vi "general_testing.vi"() -> ()   [LabVIEW 2020]
uses:
  C:/Users/359167/Documents/LabVIEW_ws/Thorlabs.MotionControl.FTD2xx_Net.dll
  Thorlabs.MotionControl.FTD2xx_Net.dll
  <vilib>/DAQmx/create/channels.llb/DAQmx Create Channel (AI-Voltage-Basic).vi
  <vilib>/Utility/file.llb/Read Delimited Spreadsheet (DBL).vi
  <vilib>/Utility/file.llb/Write Delimited Spreadsheet (DBL).vi
  <resource>/objmgr/daqmx.rc
panel:
  out "Numeric 4":dbl
  in  "Numeric 3":dbl format="%#_13g"
  out "Numeric 2":dbl
  out "appended array":dbl[](array[numeric])
  in  "y":dbl
  out "all rows":dbl[][](array[numeric])
  in  "stop":bool
  out "Numeric":i16
  in  "Y":bool[](array[boolean])
  in  "X":bool[](array[boolean])
  out "Array":refnum<k21>[][](array[refnum])
  in  "input terminal configuration":i32(ring)=-1 items=["Default"=-1, "RSE"=10083, "NRSE"=10078, "Differential"=10106, "Pseudodifferential"=12529]
  in  "Cluster":T1
  out "mounts":string[](array[string])
  out "# of mounts":dbl
  in  "# of Channels":i32=4
  out "Y":dbl[](array[numeric])
  out "X":dbl[](array[numeric])
  out "Serial Number":string[](array[string])
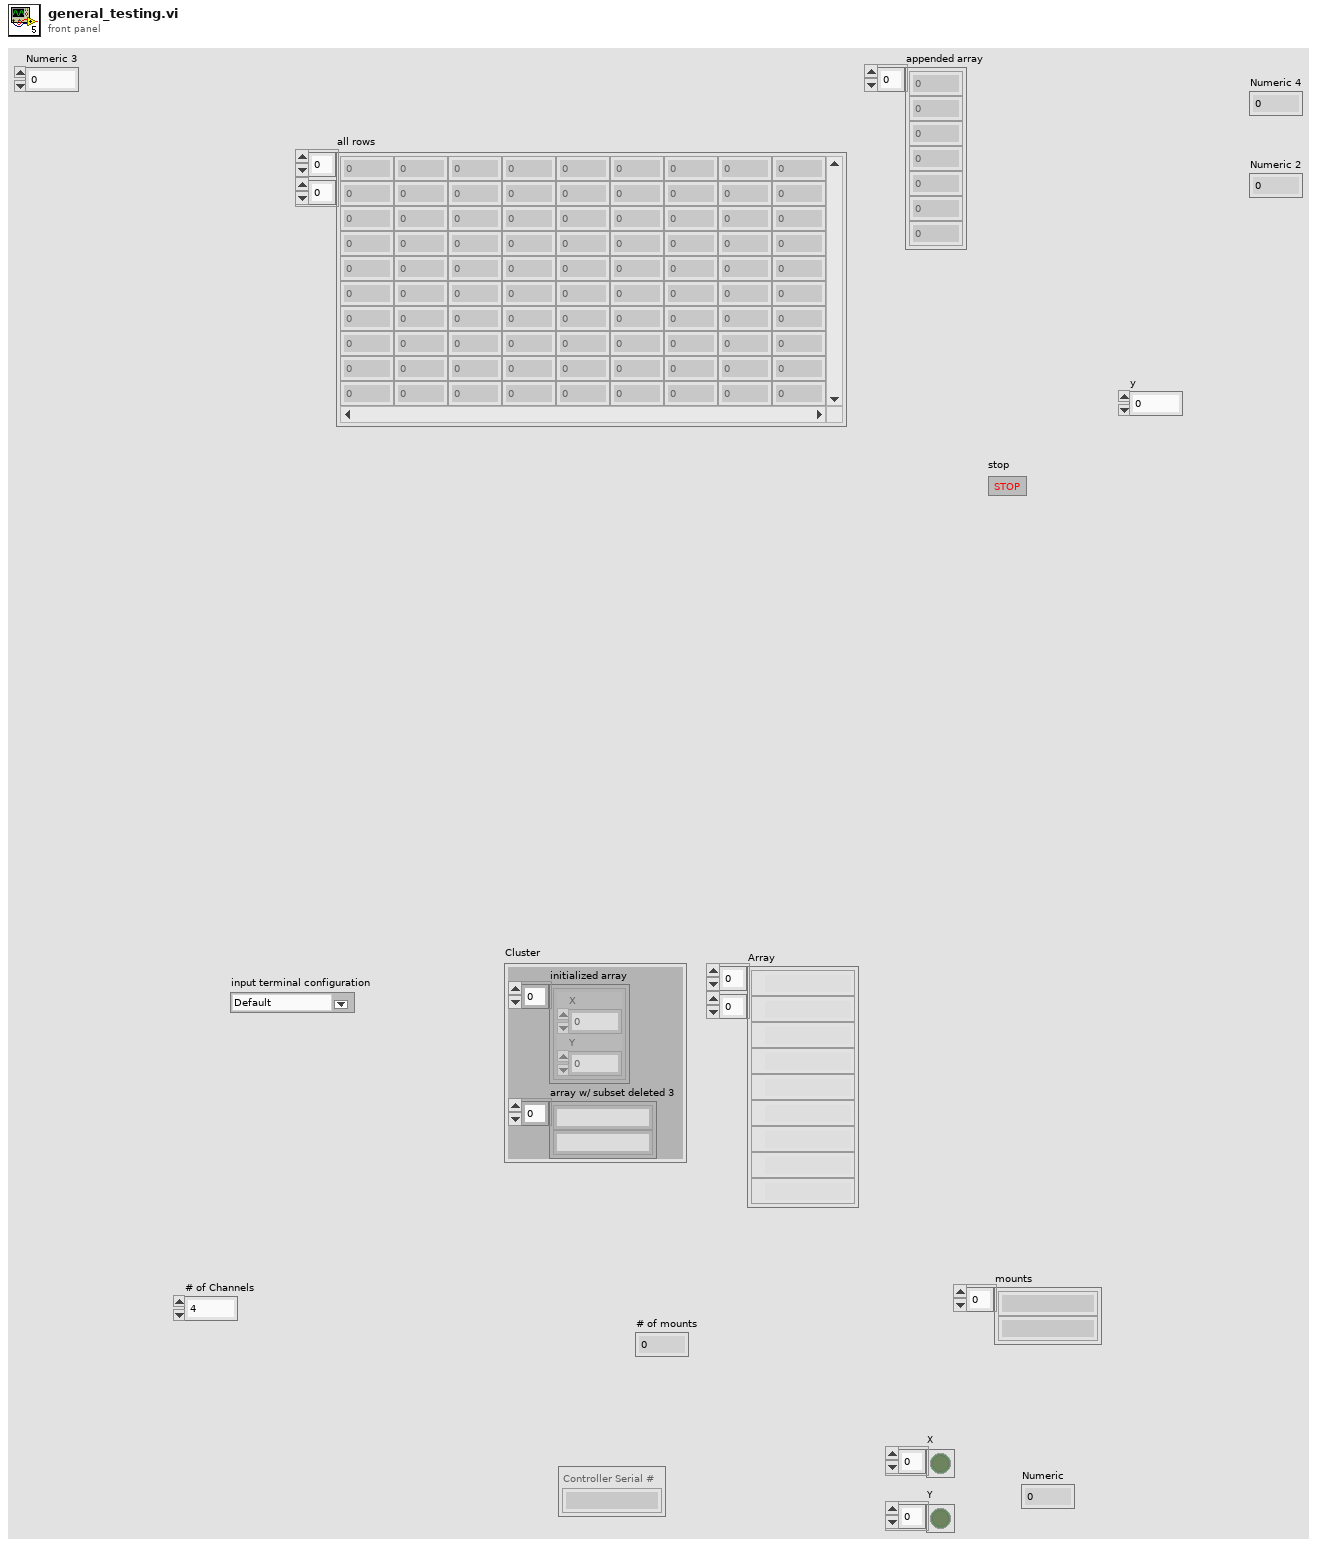
[diagram p1: front panel]
types:
  T1 = cluster{"initialized array":cluster{"X":dbl, "Y":dbl}[], "array w/ subset deleted 3":string[]}
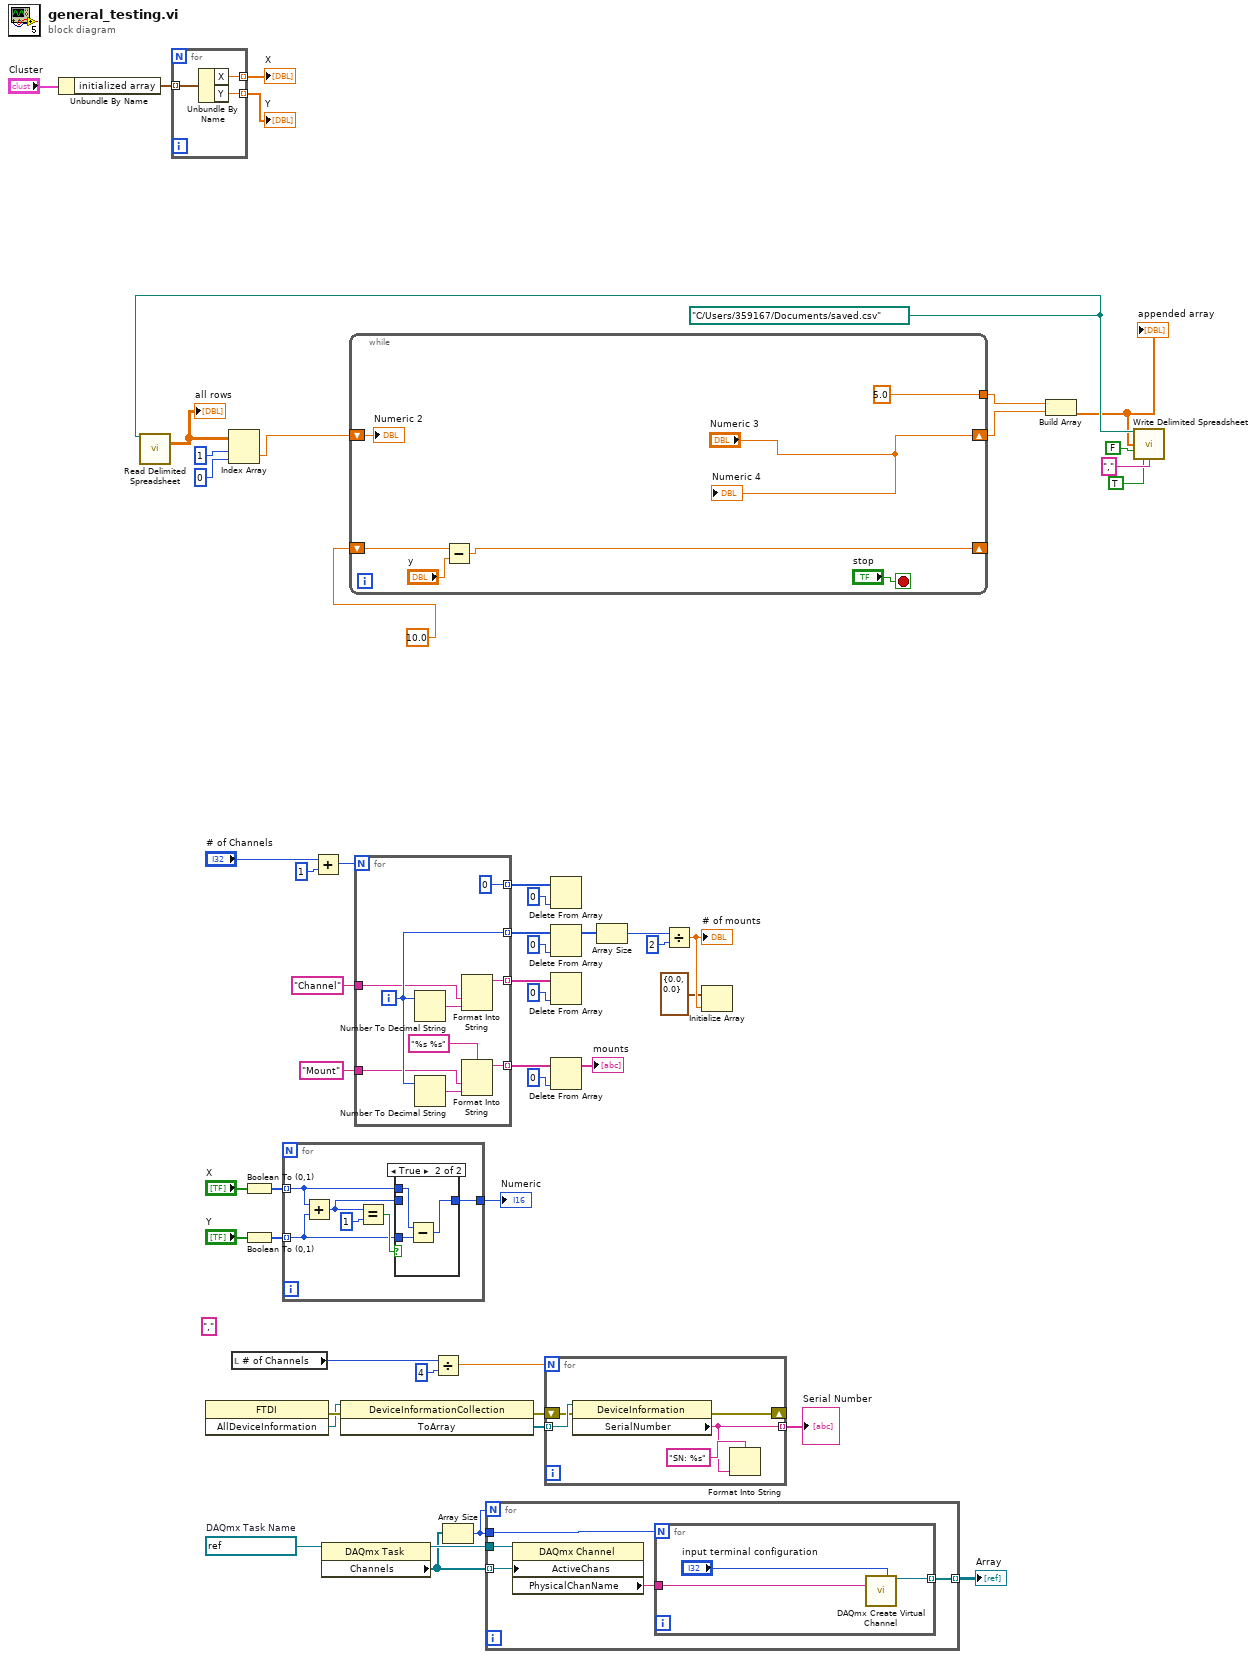
[diagram p0: block diagram]
diagram:
  w7 = path "C:/Users/359167/Documents/saved.csv" ("Path")
  (unwired) "," ("delimiter (\\t)")
  w27 = refnum<k21> "VoltageTask"  # DAQmx Task Name
  n1 = Unbundle By Name("Cluster") -> ("initialized array"=w32:cluster{"X":dbl, "Y":dbl}[])
  n2 = call-poly <vilib>:"Read Delimited Spreadsheet.vi"("file path (dialog if empty)"=w7) -> ("all rows"=w10:dbl[][])  [unwired: 9 in, 5 out]
  "all rows" <- w10
  n3 = for {
    tunnel: [w56] -> w36 mode=indexing
    tunnel: [w55] -> w35 mode=indexing
    tunnel: w32 -> [w54] mode=indexing
    n4 = Unbundle By Name(w54) -> ("X"=w56:dbl, "Y"=w55:dbl)
  }
  "X" <- w36
  "Y" <- w35
  n5 = invoke class="FTDI" method="AllDeviceInformation"() -> (error out=w44:errorcluster, "AllDeviceInformation"=w42:refnum<k24>)  [unwired: 3 in, 1 out]
  n6 = Index Array(array=w10, index (row)=1, index (col)=0 ("disabled index (col)")) -> (element=w1:dbl)
  n7 = local read "# of Channels"() -> (w37:i32)
  n8 = Boolean To (0,1)(Boolean="X") -> (0, 1=w21:i16[])
  n9 = Boolean To (0,1)(Boolean="Y") -> (0, 1=w20:i16[])
  n10 = for {
    tunnel: w21 -> [w57] mode=indexing
    tunnel: w20 -> [w58] mode=indexing
    tunnel: [w59] -> w19
    n11 = Add(x=w57, y=w58) -> (x+y=w60:i16)
    n12 = Equal?(x=w60, y=i16 1) -> (x = y?=w61:bool)
    n13 = case shown="True" w61 {
      tunnel: [w63 w64] -> w59
      tunnel: w60 -> [w63 _]
      tunnel: w58 -> [_ w66]
      tunnel: w57 -> [_ w65]
      frame False {
      }
      frame True {
        n14 = Subtract(x=w65, y=w66) -> (x-y=w64:i16)
      }
    }
  }
  "Numeric" <- w19
  n15 = Add(x="# of Channels", y=1) -> (x+y=w53:i32)
  n16 = property class="DAQmx Task"(reference=w27) -> (reference out=w28:refnum<k21>, "Channels"=w25:refnum<k21>[])  [unwired: 1 in, 1 out]
  n17 = invoke class="DeviceInformationCollection" method="ToArray"(reference=w42, error in=w44) -> (error out=w45:errorcluster, "ToArray"=w43:refnum<k24>[])  [unwired: 1 in, 1 out]
  n18 = while {
    shift-right: [w71] -> _
    shift-left: 10.0 -> [w70]
    shift-right: ["Numeric 3"] -> w5
    shift-left: w1 -> [w67]
    tunnel: [5.0] -> w4
    stop <- "stop" stop-if-true
    n19 = Subtract(x=w70, y="y") -> (x-y=w71:dbl)
    "Numeric 2" <- w67
    "Numeric 4" <- "Numeric 3"
  }
  n20 = for {
    N: w53 -> [_]
    tunnel: [w82] -> w50 mode=indexing
    tunnel: [w75] -> w33 mode=indexing
    tunnel: "Mount" -> [w77]
    tunnel: "Channel" -> [w80]
    tunnel: [w78] -> w16 mode=indexing
    tunnel: [0] -> w14 mode=indexing
    i -> [w82]
    n21 = Number To Decimal String(number=w82) -> (decimal integer string=w79:string)  [unwired: 1 in]
    n22 = Number To Decimal String(number=w82) -> (decimal integer string=w76:string)  [unwired: 1 in]
    n23 = Format Into String(w80, w79) -> (resulting string=w78:string)  [unwired: 3 in, 1 out]
    n24 = Format Into String(format string="%s %s", w77, w76) -> (resulting string=w75:string)  [unwired: 2 in, 1 out]
  }
  n25 = Divide(x=w37, y=4) -> (x/y=w38:dbl)
  n26 = Array Size(array=w25) -> (size(s)=w24:i32)
  n27 = for {
    N: w24 -> [_]
    tunnel: w25 -> [w87] mode=indexing
    tunnel: w28 -> [w86]
    tunnel: [w84] -> w26 mode=indexing
    tunnel: w24 -> [w83]
    n28 = property class="DAQmx Channel"(reference=w86, "ActiveChans"=w87) -> ("PhysicalChanName"=w85:tag)  [unwired: 1 in, 2 out]
    n29 = for {
      N: w83 -> [_]
      tunnel: [w89] -> w84 mode=indexing
      tunnel: w85 -> [w88]
      n30 = call-poly <vilib>:"DAQmx Create Virtual Channel.vi"("input terminal configuration"="input terminal configuration", "physical channels"=w88) -> ("task out"=w89:refnum<k21>)  [unwired: 12 in, 1 out]
    }
  }
  "Array" <- w26
  n31 = for {
    N: w38 -> [_]
    tunnel: w43 -> [w95] mode=indexing
    shift-right: [w93] -> _
    shift-left: w45 -> [w94]
    tunnel: [w91] -> w41 mode=indexing
    n32 = property class="DeviceInformation"(reference=w95, error in=w94) -> (error out=w93:errorcluster, "SerialNumber"=w91:string)  [unwired: 1 out]
    n33 = Format Into String(format string="SN: %s", w91) -> ()  [unwired: 2 in, 2 out]
  }
  "Serial Number" <- w41
  n34 = Delete From Array(array=w14, index=0) -> ()  [unwired: 1 in, 2 out]
  n35 = Delete From Array(array=w50, index=0) -> (array with subset deleted=w13:i32[])  [unwired: 1 in, 1 out]
  n36 = Delete From Array(array=w16, index=0) -> ()  [unwired: 1 in, 2 out]
  n37 = Delete From Array(array=w33, index=0) -> (array with subset deleted=→"mounts":string[])  [unwired: 1 in, 1 out]
  n38 = Array Size(array=w13) -> (size(s)=w39:i32)
  n39 = Divide(x=w39, y=2) -> (x/y=w47:dbl)
  "# of mounts" <- w47
  n40 = Initialize Array(cluster{"X":dbl, "Y":dbl} {"X"=0.0, "Y"=0.0}, w47) -> ()  [unwired: 1 out]
  n41 = Build Array(w4, w5) -> (w3:dbl[])
  "appended array" <- w3
  n42 = call-poly <vilib>:"Write Delimited Spreadsheet.vi"("file path (dialog if empty)"=w7, "1D data"=w3, "append to file? (new file:F)"=FALSE, "transpose? (no:F)"=TRUE, "delimiter (\\t)"="," ("delimiter (\\t)")) -> ()  [unwired: 9 in, 2 out]
